vi "comm wait for string pattern.vi"(0 "Comm Handle":u32, 1 "timeout (10000)":u32=10000, 3 "Loop Delay (10)":u32=10, 5 "match pattern":string, 7 "rx only one byte per loop (T)":bool=TRUE, 9 "string in (\"\")":string, 11 "error in (no error)":errorcluster) -> (4 "dup Comm Handle":u32, 6 "match":bool, 10 "match substring":string, 12 "before match":string, 14 "after match":string, 15 "error out":errorcluster)   [LabVIEW 2017, in "lvserial.lvlib"]
doc: "This VI is receiving the data from the device and compares the data with the string in 'pattern'. If the pattern matches, the VI returns 'match'=TRUE.\nAfter 'timeout' the 'match' is FALSE and all received data are lost.\n\nThe comparison is done by using the Match Pattern function of LabVIEW."
uses:
  lvserial.lvlib
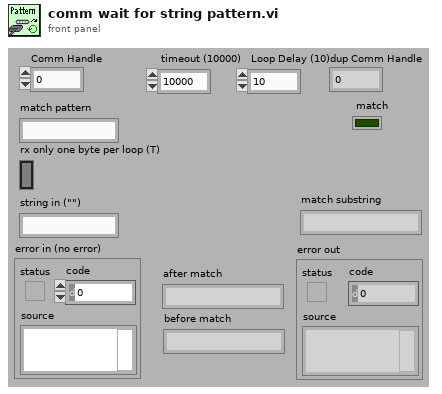
[diagram p1: front panel]
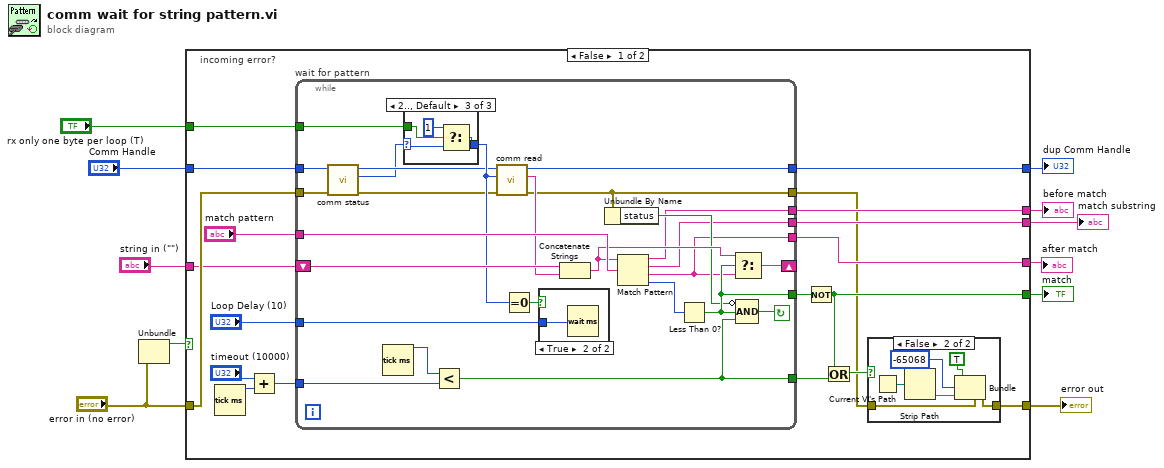
[diagram p0: block diagram]
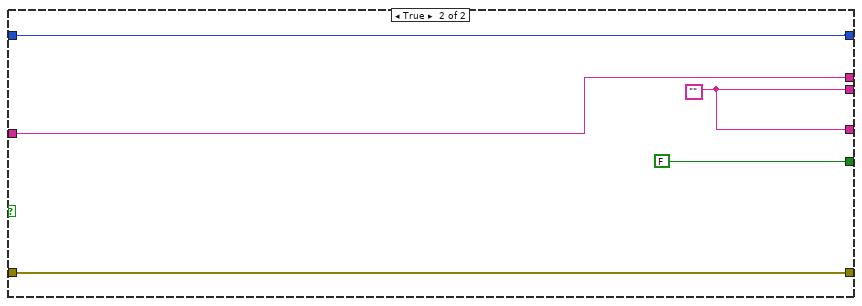
[diagram p6: hidden frame]
diagram:
  n1 = Unbundle("error in (no error)") -> ("status"=w10:bool)  [unwired: 2 out]
  n2 = case "incoming error?" shown="False" w10 {
    tunnel: [w15 FALSE] -> w11
    tunnel: "error in (no error)" -> [w20 w75]
    tunnel: [w12 w75] -> w2
    tunnel: "Comm Handle" -> [w28 w71]
    tunnel: [w25 w71] -> w1
    tunnel: [w23 w73] -> w8
    tunnel: [w22 w72] -> w7
    tunnel: [w21 w73] -> w6
    tunnel: "rx only one byte per loop (T)" -> [w19 _]
    tunnel: "string in (\"\")" -> [w18 w72]
    frame False {
      n3 = Tick Count (ms)() -> (millisecond timer value=w27:u32)
      n4 = Add(x="timeout (10000)", y=w27) -> (x+y=w29:u32)
      n5 = while "wait for pattern" {
        tunnel: w19 -> [w41]
        tunnel: [w31] -> w13
        tunnel: w20 -> [w35]
        tunnel: [w42] -> w21
        tunnel: [w43] -> w22
        tunnel: [w44] -> w23
        tunnel: "Loop Delay (10)" -> [w45]
        tunnel: [w47] -> w17
        tunnel: [w39] -> w25
        tunnel: [w48] -> w16
        tunnel: w28 -> [w36]
        tunnel: "match pattern" -> [w54]
        shift-left: w18 -> [w51]
        shift-right: [w52] -> _
        tunnel: w29 -> [w55]
        stop <- w49 continue-if-true
        n6 = call "comm status.vi"("error in (no error)"=w35, "Comm Handle"=w36) -> ("error out"=w34:errorcluster, "In Queue"=w32:u32, "dup Comm Handle"=w33:u32)  [unwired: 7 out]
        n7 = Tick Count (ms)() -> (millisecond timer value=w56:u32)
        n8 = case shown="2.., Default" w32 {
          selector: w32 -> [w58 w59 w63]
          tunnel: [w58 w59 w62] -> w38
          tunnel: w41 -> [_ _ w61]
          frame 0 {
          }
          frame 1 {
          }
          frame 2.., Default {
            n9 = Select(t=u32 1, s=w61, f=w63) -> (s? t:f=w62:u32)
          }
        }
        n10 = Less?(x=w56, y=w55) -> (x < y?=w47:bool)
        n11 = call "comm read.vi"("error in (no error)"=w34, "requested byte count"=w38, "Comm Handle"=w33) -> ("error out"=w31:errorcluster, "string read"=w37:string, "dup Comm Handle"=w39:u32)  [unwired: 6 out]
        n12 = Equal To 0?(x=w38) -> (x = 0?=w40:bool)
        n13 = case shown="True" w40 {
          tunnel: w45 -> [_ w57]
          frame False {
          }
          frame True {
            n14 = Wait (ms)(milliseconds to wait=w57) -> ()  [unwired: 1 out]
          }
        }
        n15 = Concatenate Strings(w51, w37) -> (w50:string)
        n16 = Unbundle By Name(w31) -> ("status"=w46:bool)
        n17 = Match Pattern(string=w50, regular expression=w54) -> (before substring=w43:string, match substring=w42:string, after substring=w44:string, offset past match=w53:i32)  [unwired: 1 out]
        n18 = Less Than 0?(x=w53) -> (x < 0?=w48:bool)
        n19 = Select(t=w50, s=w48, f=w44) -> (s? t:f=w52:string)
        n20 = Compound Arithmetic op=AND(invert w46, w48, w47) -> (w49:bool)
      }
      n21 = Not(x=w16) -> (.not. x?=w15:bool)
      n22 = Or(x=w15, y=w17) -> (x .or. y?=w14:bool)
      n23 = case shown="False" w14 {
        tunnel: w13 -> [w64 w70]
        tunnel: [w64 w69] -> w12
        frame True {
        }
        frame False {
          n24 = Current VI's Path() -> (path=w66:path)
          n25 = Strip Path(path=w66) -> (name=w67:string)  [unwired: 1 out]
          n26 = Bundle(cluster=w70, "status"=TRUE, "code"=-65068, "source"=w67) -> (w69:errorcluster)
        }
      }
    }
    frame True {
      w73 = ""
    }
  }
  "match" <- w11
  "dup Comm Handle" <- w1
  "after match" <- w8
  "before match" <- w7
  "match substring" <- w6
  "error out" <- w2
